vi "Make Error.vi"(8 "error in (no error)":errorcluster, 11 "DigitiserActor in":refnum<class "DigitiserActor.lvclass">) -> (0 "error out":errorcluster, 3 "DigitiserActor out":refnum<class "DigitiserActor.lvclass">)   [LabVIEW 2019, in "DigitiserActor.lvlib" / "DigitiserActor.lvclass"]
uses:
  DigitiserActor.lvclass
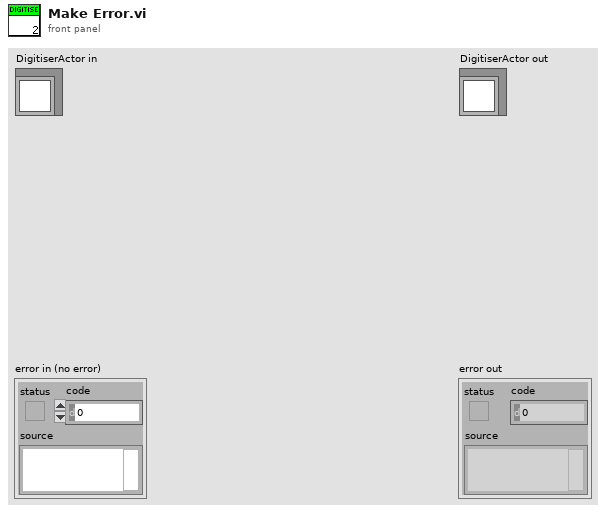
[diagram p1: front panel]
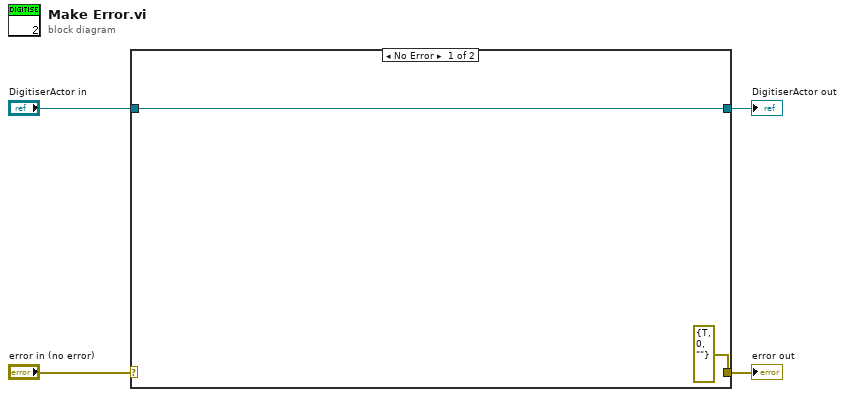
[diagram p0: block diagram]
diagram:
  n1 = case shown="No Error" "error in (no error)" {
    selector: "error in (no error)" -> [_ w8]
    tunnel: [errorcluster {"status"=TRUE, "code"=0, "source"=""} ("error IO") w8] -> w3
    tunnel: [w6 w7] -> w1
    tunnel: "DigitiserActor in" -> [w6 w7]
    frame No Error {
    }
    frame Error {
    }
  }
  "error out" <- w3
  "DigitiserActor out" <- w1
